vi "confirm_popup_only_warning.vi"(5 "Warning(T)/Inf(F)":bool, 7 "Title":string, 8 "error_in":errorcluster, 9 "True Label":string, 11 "Message":string) -> (0 "error_out":errorcluster, 3 "Result":bool)   [LabVIEW 2020]
uses:
  AULocalize/SubVIs/Get Localized Phrase Compact Interface 0D.vi
panel:
  out "Project Title 2":string
  out "Message copy":string
  in  "True":bool
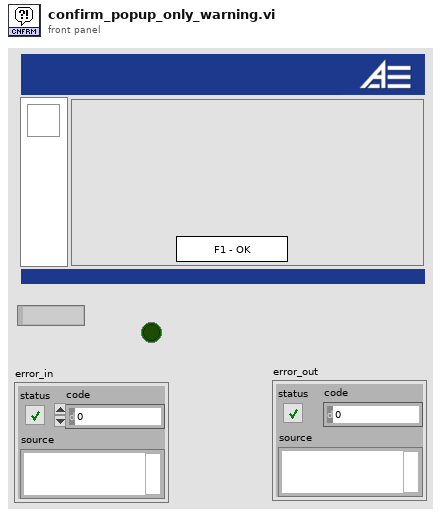
[diagram p1: front panel]
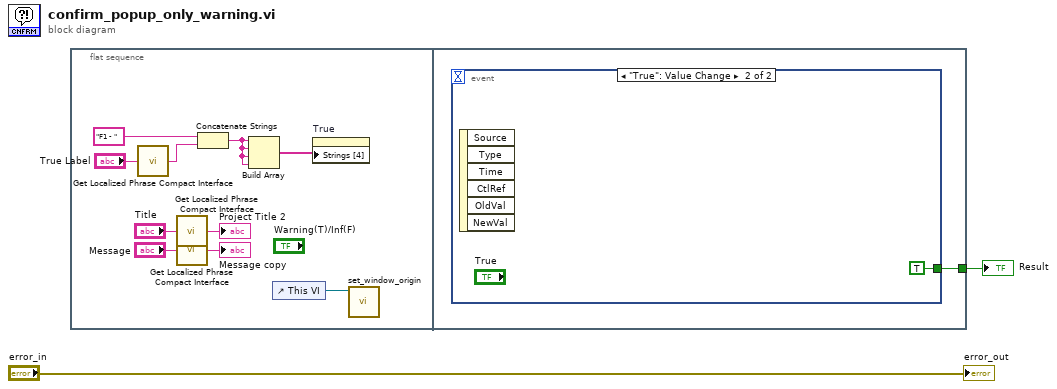
[diagram p0: block diagram]
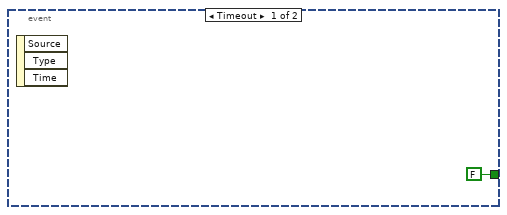
[diagram p2: hidden frame]
diagram:
  n1 = flat-sequence {
    tunnel: [w13] -> w2
    frame #0 {
      n2 = call-poly "Get Localized Phrase Compact Interface.vi"("Key"="True Label") -> ("Translated Phrase"=w5:string)
      n3 = call-poly "Get Localized Phrase Compact Interface.vi"("Key"="Title") -> ("Translated Phrase"=→"Project Title 2":string)
      n4 = call-poly "Get Localized Phrase Compact Interface.vi"("Key"="Message") -> ("Translated Phrase"=→"Message copy":string)
      n5 = Concatenate Strings("F1 - ", w5) -> (w7:string)
      n6 = Build Array(w7, w7, w7, w7) -> (w10:string[])
      n7 = control-ref of="This VI"() -> (w6:refnum<vi>)
      n8 = property on="True" class="Bool"("Strings [4]"=w10) -> ()  [unwired: 2 in, 2 out]
      n9 = call "set_window_origin.vi"("this_vi_reference"=w6) -> ()  [unwired: 10 in, 1 out]
    }
    frame #1 {
      n10 = event shown="[1] \"True\": Value Change" {
        selector: _ -> [_ _]
        dyn-events: _ -> [_ _]
        timeout: _ -> [_ _]
        tunnel: [FALSE TRUE] -> w13
        event Timeout {
          n11 = event-data() -> ()  [unwired: 1 in, 3 out]
        }
        event "True": Value Change {
          n12 = event-data() -> ()  [unwired: 1 in, 6 out]
        }
      }
    }
  }
  "Result" <- w2
  "error_out" <- "error_in"
